vi "功能试验判定.vi"(7 "Result":refnum<vi>, 10 "判定参数":T1, 11 "XY曲线":cluster{"X":dbl[], "Y":dbl[]}[](array[cluster])) -> (2 "判定项长度":i32, 3 "OK？":bool)   [LabVIEW 2019]
uses:
  <userlib>/_MGI/1D Array/MGI Average/MGI Average (DBL[]).vi
panel:
  out "逆向平均值":dbl
  out "正向平均值":dbl
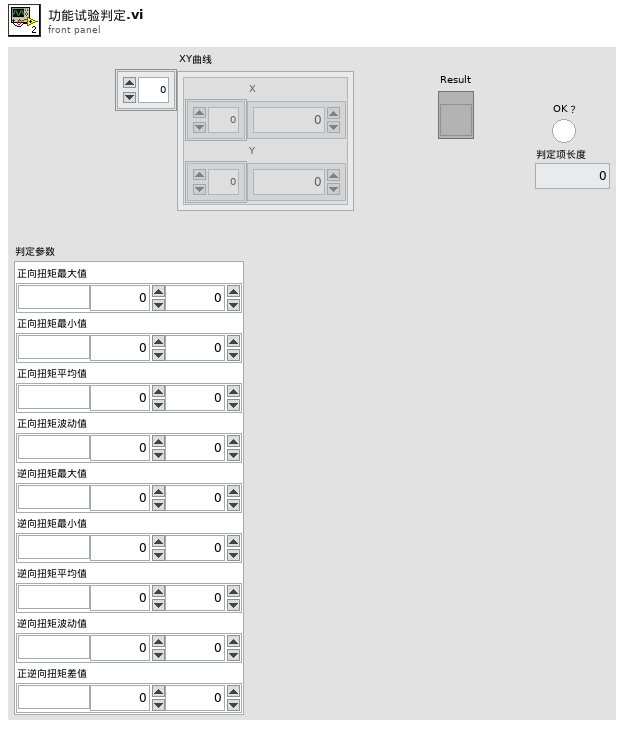
[diagram p1: front panel]
types:
  T1 = cluster{"正向扭矩最大值":cluster{"单位":string, "下限":dbl, "上限":dbl}, "正向扭矩最小值":cluster{"单位":string, "下限":dbl, "上限":dbl}, "正向扭矩平均值":cluster{"单位":string, "下限":dbl, "上限":dbl}, "正向扭矩波动值":cluster{"单位":string, "下限":dbl, "上限":dbl}, "逆向扭矩最大值":cluster{"单位":string, "下限":dbl, "上限":dbl}, "逆向扭矩最小值":cluster{"单位":string, "下限":dbl, "上限":dbl}, "逆向扭矩平均值":cluster{"单位":string, "下限":dbl, "上限":dbl}, "逆向扭矩波动值":cluster{"单位":string, "下限":dbl, "上限":dbl}, "正逆向扭矩差值":cluster{"单位":string, "下限":dbl, "上限":dbl}}
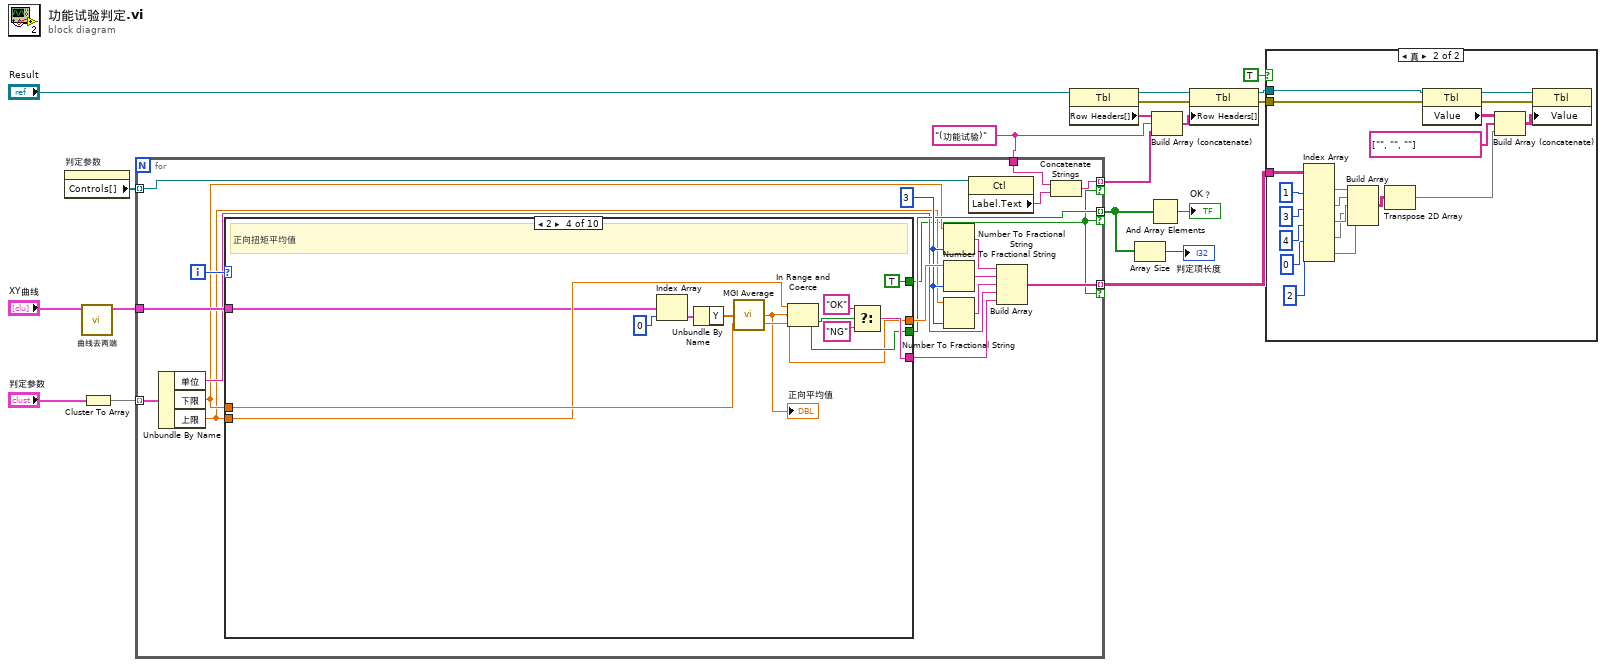
[diagram p0: block diagram]
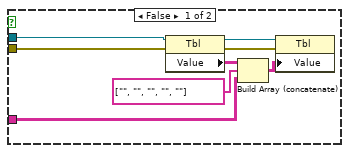
[diagram p2: hidden frame]
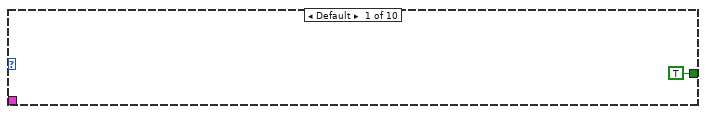
[diagram p3: hidden frame]
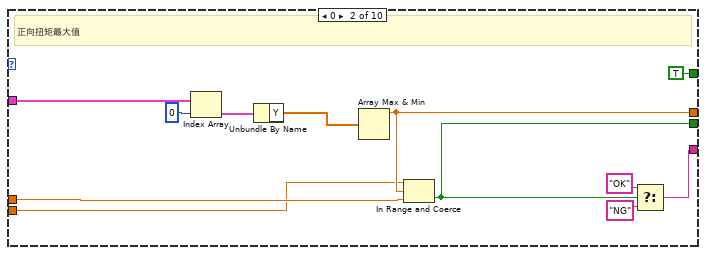
[diagram p4: hidden frame]
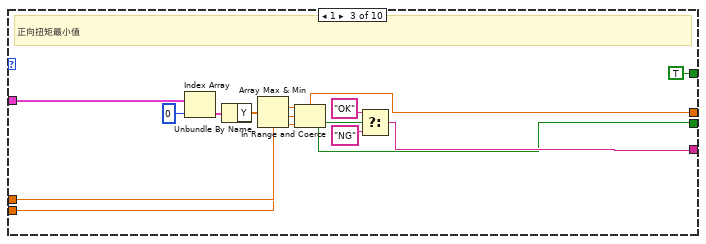
[diagram p5: hidden frame]
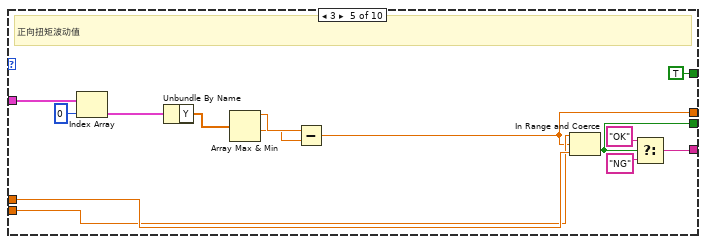
[diagram p6: hidden frame]
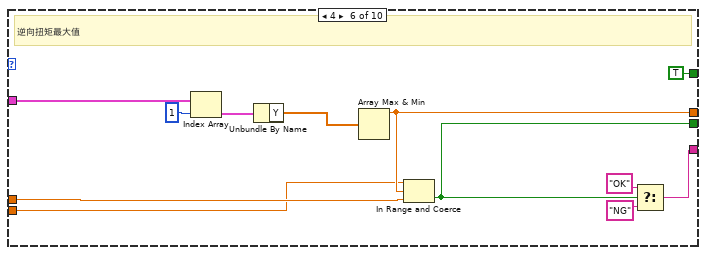
[diagram p7: hidden frame]
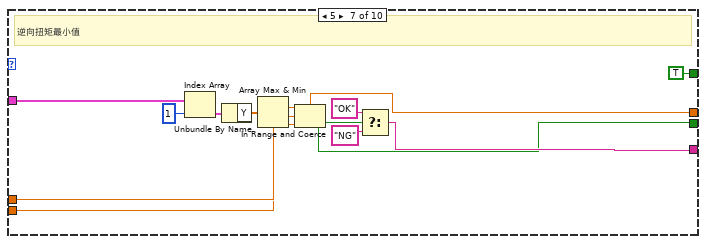
[diagram p8: hidden frame]
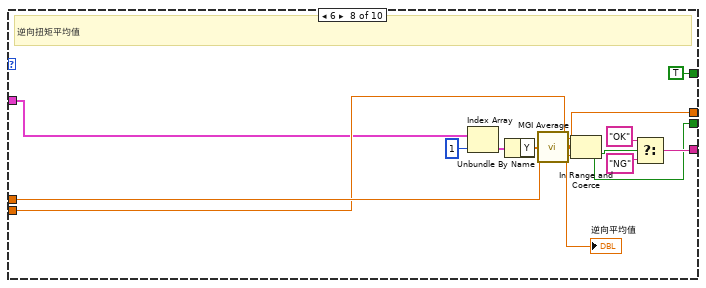
[diagram p9: hidden frame]
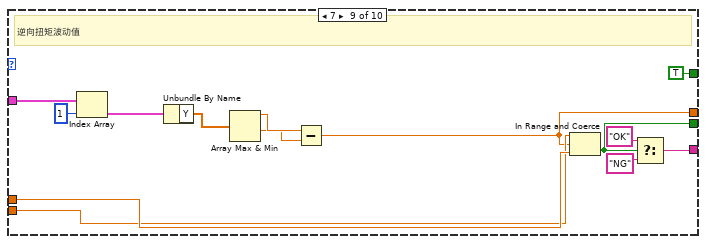
[diagram p10: hidden frame]
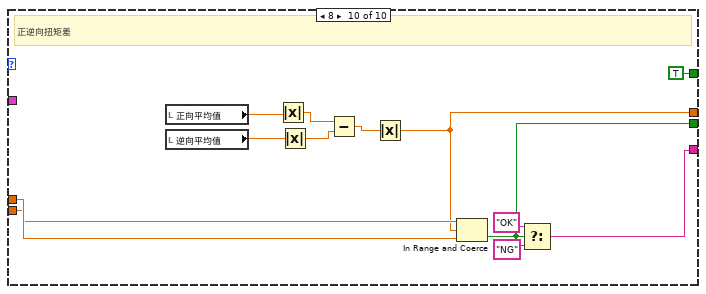
[diagram p11: hidden frame]
diagram:
  w1 = "(功能试验)" ("Label.Text")
  n1 = property on="判定参数" class="Clust (严格)"() -> ("Controls[]"=w8:refnum<vi>[])  [unwired: 2 in, 2 out]
  n2 = call "曲线去两端.vi"("曲线In"="XY曲线") -> ("曲线Out"=w4:cluster{"X":dbl[], "Y":dbl[]}[])  [unwired: 9 in, 1 out]
  n3 = Cluster To Array(cluster="判定参数") -> (array=w19:cluster{"单位":string, "下限":dbl, "上限":dbl}[])
  n4 = for {
    tunnel: w19 -> [w38] mode=indexing
    tunnel: w8 -> [w36] mode=indexing
    tunnel: w4 -> [w34]
    tunnel: [w28] -> w3 mode=indexing if=w23
    tunnel: [w24] -> w9 mode=indexing if=w23
    tunnel: [w20] -> w12 mode=indexing if=w23
    tunnel: w1 -> [w21]
    i -> [w37]
    w33 = i16 3 ("精度(6)")
    n5 = Unbundle By Name(w38) -> ("单位"=w27:string, "下限"=w26:dbl, "上限"=w25:dbl)
    n6 = case shown="2" w37 {
      tunnel: [_ w48 w54 w64 w76 w98 w104 w114 w126 w140] -> w35
      tunnel: w34 -> [_ w51 w63 w68 w82 w101 w113 w118 w132 _]
      tunnel: [_ w45 w59 w73 w87 w95 w109 w123 w137 w142] -> w29
      tunnel: [_ w44 w58 w72 w86 w94 w108 w122 w136 w141] -> w28
      tunnel: w26 -> [_ w43 w57 w71 w85 w93 w107 w121 w135 w149]
      tunnel: w25 -> [_ w42 w56 w70 w84 w92 w106 w120 w134 w148]
      tunnel: [TRUE TRUE TRUE TRUE TRUE TRUE TRUE TRUE TRUE TRUE] -> w23
      frame Default {
      }
      frame 0 {
        # "正向扭矩最大值"
        n7 = Index Array(array=w51, index=0 ("索引")) -> (element=w49:cluster{"X":dbl[], "Y":dbl[]})
        n8 = Unbundle By Name(w49) -> ("Y"=w40:dbl[])
        n9 = Array Max & Min(array=w40) -> (max value=w48:dbl)  [unwired: 3 out]
        n10 = In Range and Coerce(upper limit=w42, x=w48, lower limit=w43) -> (In Range?=w44:bool)  [unwired: 1 out]
        n11 = Select(t="OK", s=w44, f="NG") -> (s? t:f=w45:string)
      }
      frame 1 {
        # "正向扭矩最小值"
        n12 = Index Array(array=w63, index=0 ("索引")) -> (element=w62:cluster{"X":dbl[], "Y":dbl[]})
        n13 = Unbundle By Name(w62) -> ("Y"=w53:dbl[])
        n14 = Array Max & Min(array=w53) -> (min value=w54:dbl)  [unwired: 3 out]
        n15 = In Range and Coerce(upper limit=w56, x=w54, lower limit=w57) -> (In Range?=w58:bool)  [unwired: 1 out]
        n16 = Select(t="OK", s=w58, f="NG") -> (s? t:f=w59:string)
      }
      frame 2 {
        # "正向扭矩平均值"
        n17 = Index Array(array=w68, index=0 ("索引")) -> (element=w67:cluster{"X":dbl[], "Y":dbl[]})
        n18 = Unbundle By Name(w67) -> ("Y"=w66:dbl[])
        n19 = call-poly <userlib>:"MGI Average.vi"("Double[]"=w66) -> ("Average"=w64:dbl)  [unwired: 1 in]
        "正向平均值" <- w64
        n20 = In Range and Coerce(upper limit=w70, x=w64, lower limit=w71) -> (In Range?=w72:bool)  [unwired: 1 out]
        n21 = Select(t="OK", s=w72, f="NG") -> (s? t:f=w73:string)
      }
      frame 3 {
        # "正向扭矩波动值"
        n22 = Index Array(array=w82, index=0 ("索引")) -> (element=w81:cluster{"X":dbl[], "Y":dbl[]})
        n23 = Unbundle By Name(w81) -> ("Y"=w79:dbl[])
        n24 = Array Max & Min(array=w79) -> (max value=w78:dbl, min value=w77:dbl)  [unwired: 2 out]
        n25 = Subtract(x=w78, y=w77) -> (x-y=w76:dbl)
        n26 = In Range and Coerce(upper limit=w84, x=w76, lower limit=w85) -> (In Range?=w86:bool)  [unwired: 1 out]
        n27 = Select(t="OK", s=w86, f="NG") -> (s? t:f=w87:string)
      }
      frame 4 {
        # "逆向扭矩最大值"
        n28 = Index Array(array=w101, index=1 ("索引")) -> (element=w99:cluster{"X":dbl[], "Y":dbl[]})
        n29 = Unbundle By Name(w99) -> ("Y"=w90:dbl[])
        n30 = Array Max & Min(array=w90) -> (max value=w98:dbl)  [unwired: 3 out]
        n31 = In Range and Coerce(upper limit=w92, x=w98, lower limit=w93) -> (In Range?=w94:bool)  [unwired: 1 out]
        n32 = Select(t="OK", s=w94, f="NG") -> (s? t:f=w95:string)
      }
      frame 5 {
        # "逆向扭矩最小值"
        n33 = Index Array(array=w113, index=1 ("索引")) -> (element=w112:cluster{"X":dbl[], "Y":dbl[]})
        n34 = Unbundle By Name(w112) -> ("Y"=w103:dbl[])
        n35 = Array Max & Min(array=w103) -> (min value=w104:dbl)  [unwired: 3 out]
        n36 = In Range and Coerce(upper limit=w106, x=w104, lower limit=w107) -> (In Range?=w108:bool)  [unwired: 1 out]
        n37 = Select(t="OK", s=w108, f="NG") -> (s? t:f=w109:string)
      }
      frame 6 {
        # "逆向扭矩平均值"
        n38 = Index Array(array=w118, index=1 ("索引")) -> (element=w117:cluster{"X":dbl[], "Y":dbl[]})
        n39 = Unbundle By Name(w117) -> ("Y"=w116:dbl[])
        n40 = call-poly <userlib>:"MGI Average.vi"("Double[]"=w116) -> ("Average"=w114:dbl)  [unwired: 1 in]
        "逆向平均值" <- w114
        n41 = In Range and Coerce(upper limit=w120, x=w114, lower limit=w121) -> (In Range?=w122:bool)  [unwired: 1 out]
        n42 = Select(t="OK", s=w122, f="NG") -> (s? t:f=w123:string)
      }
      frame 7 {
        # "逆向扭矩波动值"
        n43 = Index Array(array=w132, index=1 ("索引")) -> (element=w131:cluster{"X":dbl[], "Y":dbl[]})
        n44 = Unbundle By Name(w131) -> ("Y"=w129:dbl[])
        n45 = Array Max & Min(array=w129) -> (max value=w128:dbl, min value=w127:dbl)  [unwired: 2 out]
        n46 = Subtract(x=w128, y=w127) -> (x-y=w126:dbl)
        n47 = In Range and Coerce(upper limit=w134, x=w126, lower limit=w135) -> (In Range?=w136:bool)  [unwired: 1 out]
        n48 = Select(t="OK", s=w136, f="NG") -> (s? t:f=w137:string)
      }
      frame 8 {
        # "正逆向扭矩差"
        n49 = local read "正向平均值"() -> (w147:dbl)
        n50 = local read "逆向平均值"() -> (w146:dbl)
        n51 = Absolute Value(x=w147) -> (abs(x)=w145:dbl)
        n52 = Absolute Value(x=w146) -> (abs(x)=w144:dbl)
        n53 = Subtract(x=w145, y=w144) -> (x-y=w143:dbl)
        n54 = Absolute Value(x=w143) -> (abs(x)=w140:dbl)
        n55 = In Range and Coerce(upper limit=w148, x=w140, lower limit=w149) -> (In Range?=w141:bool)  [unwired: 1 out]
        n56 = Select(t="OK", s=w141, f="NG") -> (s? t:f=w142:string)
      }
    }
    n57 = Number To Fractional String(number=w26, precision (6)=w33) -> (F-format string=w32:string)  [unwired: 2 in]
    n58 = Number To Fractional String(number=w35, precision (6)=w33) -> (F-format string=w31:string)  [unwired: 2 in]
    n59 = Number To Fractional String(number=w25, precision (6)=w33) -> (F-format string=w30:string)  [unwired: 2 in]
    n60 = property class="Ctl"(reference=w36) -> ("Label.Text"=w22:string)  [unwired: 1 in, 2 out]
    n61 = Build Array(w32, w31, w30, w27, w29) -> (w24:string[])
    n62 = Concatenate Strings(w21, w22) -> (w20:string)
  }
  n63 = property class="Tbl"(reference="Result") -> (reference out=w14:refnum<vi>, error out=w17:errorcluster, "Row Headers[]"=w10:string[])  [unwired: 1 in]
  n64 = Array Size(array=w3) -> (size(s)=→"判定项长度":i32)
  n65 = And Array Elements(Boolean array=w3) -> (logical AND=→"OK？":bool)
  n66 = Build Array (concatenate)(w10, w1, w12) -> (w13:string[])
  n67 = property class="Tbl"(reference=w14, error in=w17, "Row Headers[]"=w13) -> (reference out=w15:refnum<vi>, error out=w16:errorcluster)
  n68 = case shown="真" TRUE {
    tunnel: w16 -> [w158 w178]
    tunnel: w15 -> [w155 w175]
    tunnel: w9 -> [w154 w166]
    frame False {
      n69 = property class="Tbl"(reference=w155, error in=w158) -> (reference out=w156:refnum<vi>, error out=w157:errorcluster, "Value"=w159:string[][])
      n70 = Build Array (concatenate)(w159, string[] ["", "", "", "", ""], w154) -> (w160:string[][])
      n71 = property class="Tbl"(reference=w156, error in=w157, "Value"=w160) -> ()  [unwired: 2 out]
    }
    frame True {
      n72 = Index Array(array=w166, index (col) #1=1 ("禁用的索引 (列)"), index (col) #2=3 ("索引 (列)"), index (col) #3=4 ("索引 (列)"), index (col) #4=0 ("索引 (列)"), index (col) #5=2 ("索引 (列)")) -> (element #1=w170:string[], element #2=w171:string[], element #3=w172:string[], element #4=w162:string[], element #5=w161:string[])  [unwired: 5 in]
      n73 = Build Array(w170, w171, w172, w162, w161) -> (w173:string[][])
      n74 = Transpose 2D Array(2D array=w173) -> (transposed array=w165:string[][])
      n75 = property class="Tbl"(reference=w175, error in=w178) -> (reference out=w176:refnum<vi>, error out=w177:errorcluster, "Value"=w179:string[][])
      n76 = Build Array (concatenate)(w179, string[] ["", "", ""], w165) -> (w180:string[][])
      n77 = property class="Tbl"(reference=w176, error in=w177, "Value"=w180) -> ()  [unwired: 2 out]
    }
  }
